vi "Weather Simulator.vi"() -> ()   [LabVIEW 2023]
doc: "The main VI for the Weather Monitor Simulator built application. This VI simulates weather data and puts the simulated data into the Weather Monitor data store, which allows the included web service to access the data."
uses:
  Weather Data.ctl
  Weather Data.lvlib
panel:
  in  "Enable CORS":bool
  in  "Update interval":i32=1000
  out "Wind Direction":dbl
  out "Wind Speed":dbl
  out "Pressure":dbl
  out "Temperature":dbl
  in  "Stop":bool
  # "Overview: Demonstrates the use of Web Services in a built application to provide remote access to an application's data.\nRequirements: LabVIEW Full Development System\nInstructions:\n1. Build and run the Weather Simulator (Server) build specification.\n2. Run the Weather Monitor.vi client or build and run the Weather Monitor (Client) build specification.\n3. See README.htm for more information, including how to run this VI for debugging."
  # "Weather Data Simulator"
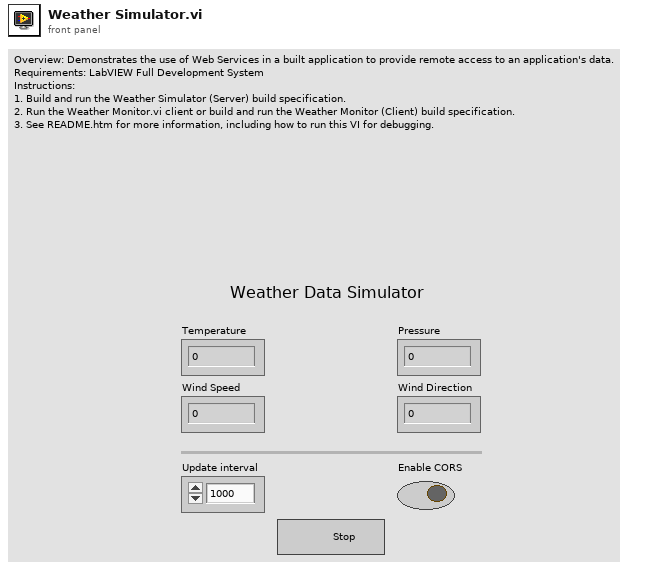
[diagram p1: front panel]
types:
  T1 = typedef "Weather Data.lvlib/Weather Data.ctl" = cluster{"Temperature":dbl, "Pressure":dbl, "Wind Speed":dbl, "Wind Direction":dbl}
  T2 = typedef "Web Service Settings.ctl" = cluster{"Enable CORS":bool}
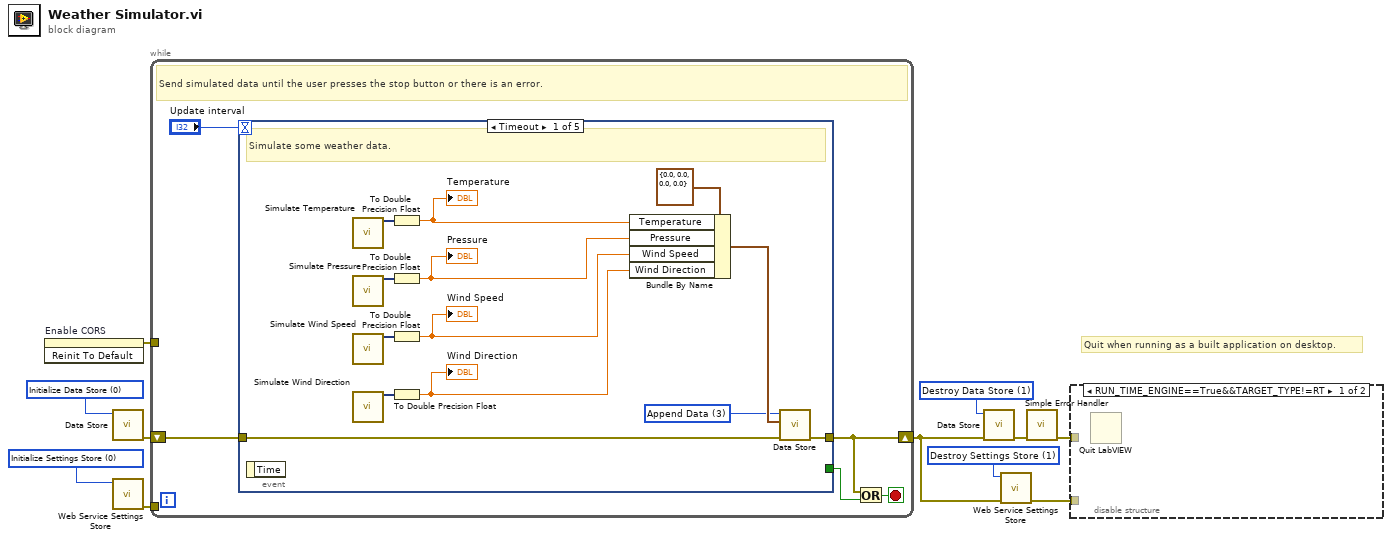
[diagram p0: block diagram]
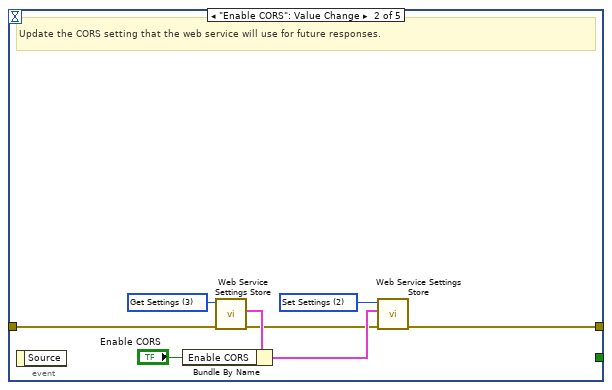
[diagram p3: hidden frame]
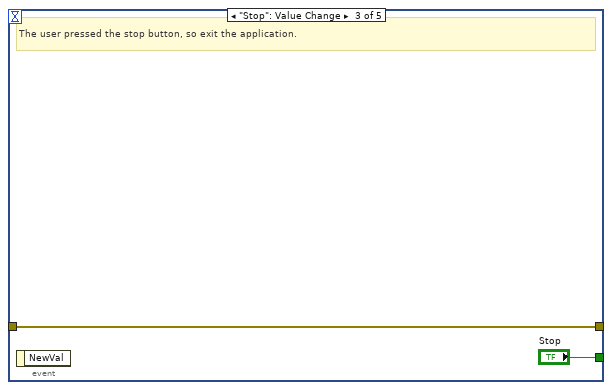
[diagram p4: hidden frame]
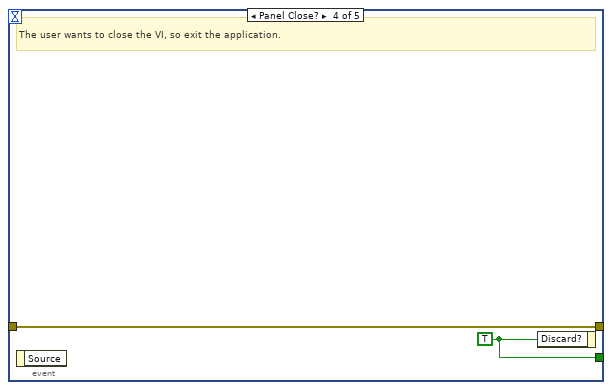
[diagram p5: hidden frame]
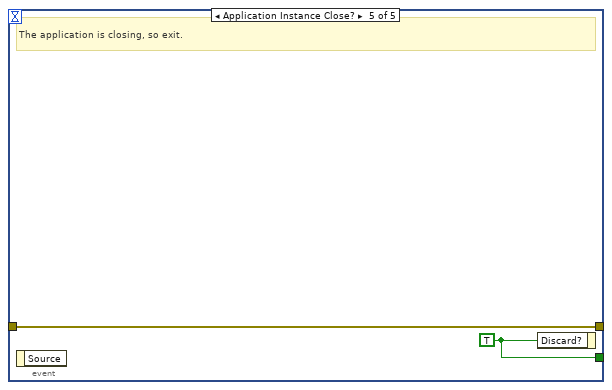
[diagram p6: hidden frame]
diagram:
  w4 = u16 1 items=["Initialize Settings Store", "Destroy Settings Store", "Set Settings", "Get Settings"] ("action")
  w6 = u16 0 items=["Initialize Settings Store", "Destroy Settings Store", "Set Settings", "Get Settings"] ("action")
  w8 = u16 1 items=["Initialize Data Store", "Destroy Data Store", "Clear Data", "Append Data", "Get Last Data", "Get All Data"] ("action")
  w10 = u16 0 items=["Initialize Data Store", "Destroy Data Store", "Clear Data", "Append Data", "Get Last Data", "Get All Data"] ("action")
  # "Quit when running as a built application on desktop."
  n1 = invoke on="Enable CORS" class="Bool (strict)" method="Reinit To Default"() -> (error out=w1:errorcluster)  [unwired: 3 in, 2 out]
  n2 = call "Data Store.vi"("action"=w10) -> ("error out"=w9:errorcluster)  [unwired: 9 in, 1 out]
  n3 = call "Web Service Settings Store.vi"("action"=w6) -> ("error out"=w5:errorcluster)  [unwired: 9 in, 1 out]
  n4 = while {
    shift-right: [w14] -> w3
    shift-left: w9 -> [w16]
    tunnel: w5 -> [_]
    tunnel: w1 -> [_]
    stop <- w15 stop-if-true
    # "Send simulated data until the user presses the stop button or there is an error."
    n5 = event shown="[0] Timeout" {
      selector: _ -> [_ _ _ _ _]
      dyn-events: _ -> [_ _ _ _ _]
      timeout: "Update interval" -> [_ _ _ _ _]
      tunnel: w16 -> [w25 w31 w39 w41 w43]
      tunnel: [w23 w30 w39 w41 w43] -> w14
      tunnel: [_ _ "Stop" w40 w42] -> w12
      event Timeout {
        w17 = u16 3 items=["Initialize Data Store", "Destroy Data Store", "Clear Data", "Append Data", "Get Last Data", "Get All Data"] ("action")
        # "Simulate some weather data."
        n6 = event-data() -> ()  [unwired: 1 in, 1 out]
        n7 = call "Simulate Temperature"() -> ("DC with Uniform Noise"=w22:dynamicdata)  [unwired: 5 in, 10 out]
        n8 = call "Simulate Pressure"() -> ("Sine with Uniform Noise"=w28:dynamicdata)  [unwired: 8 in, 7 out]
        n9 = call "Simulate Wind Speed"() -> ("Sine with Uniform Noise"=w27:dynamicdata)  [unwired: 8 in, 7 out]
        n10 = call "Simulate Wind Direction"() -> ("Sine with Uniform Noise"=w26:dynamicdata)  [unwired: 8 in, 7 out]
        n11 = To Double Precision Float(number=w22) -> (double precision float=w21:dbl)
        "Temperature" <- w21
        n12 = To Double Precision Float(number=w28) -> (double precision float=w20:dbl)
        "Pressure" <- w20
        n13 = To Double Precision Float(number=w27) -> (double precision float=w19:dbl)
        "Wind Speed" <- w19
        n14 = To Double Precision Float(number=w26) -> (double precision float=w18:dbl)
        "Wind Direction" <- w18
        n15 = Bundle By Name(cluster=T1 {"Temperature"=0.0, "Pressure"=0.0, "Wind Speed"=0.0, "Wind Direction"=0.0} ("Weather Data"), "Temperature"=w21, "Pressure"=w20, "Wind Speed"=w19, "Wind Direction"=w18) -> (w24:T1)
        n16 = call "Data Store.vi"("error in (no error)"=w25, "new weather data"=w24, "action"=w17) -> ("error out"=w23:errorcluster)  [unwired: 7 in, 1 out]
      }
      event "Enable CORS": Value Change {
        w34 = u16 2 items=["Initialize Settings Store", "Destroy Settings Store", "Set Settings", "Get Settings"] ("action")
        w37 = u16 3 items=["Initialize Settings Store", "Destroy Settings Store", "Set Settings", "Get Settings"] ("action")
        # "Update the CORS setting that the web service will use for future responses."
        n17 = event-data() -> ()  [unwired: 1 in, 1 out]
        n18 = call "Web Service Settings Store.vi"("error in (no error)"=w31, "action"=w37) -> ("error out"=w32:errorcluster, "settings out"=w36:T2)  [unwired: 8 in]
        n19 = Bundle By Name(cluster=w36, "Enable CORS"="Enable CORS") -> (w33:T2)
        n20 = call "Web Service Settings Store.vi"("error in (no error)"=w32, "new settings"=w33, "action"=w34) -> ("error out"=w30:errorcluster)  [unwired: 7 in, 1 out]
      }
      event "Stop": Value Change {
        # "The user pressed the stop button, so exit the application."
        n21 = event-data() -> ()  [unwired: 1 in, 1 out]
      }
      event Panel Close? {
        w40 = TRUE ("Discard?")
        # "The user wants to close the VI, so exit the application."
        n22 = event-data() -> ()  [unwired: 1 in, 1 out]
        n23 = event-data("Discard?"=w40) -> ()  [unwired: 1 in, 1 out]
      }
      event Application Instance Close? {
        w42 = TRUE ("Discard?")
        # "The application is closing, so exit."
        n24 = event-data() -> ()  [unwired: 1 in, 1 out]
        n25 = event-data("Discard?"=w42) -> ()  [unwired: 1 in, 1 out]
      }
    }
    n26 = Or(x=w14, y=w12) -> (x .or. y?=w15:bool)
  }
  n27 = call "Data Store.vi"("error in (no error)"=w3, "action"=w8) -> ("error out"=w11:errorcluster)  [unwired: 8 in, 1 out]
  n28 = call "Web Service Settings Store.vi"("error in (no error)"=w3, "action"=w4) -> ("error out"=w2:errorcluster)  [unwired: 8 in, 1 out]
  n29 = call <vilib>:"Simple Error Handler.vi"("error in (no error)"=w11) -> ("error out"=w7:errorcluster)  [unwired: 4 in, 4 out]
  n30 = disable-structure shown="RUN_TIME_ENGINE==True&&TARGET_TYPE!=RT" {
    disable-tunnel: w7 -> [_ _]
    disable-tunnel: w2 -> [_ _]
    frame condition #0 {
      n31 = Quit LabVIEW() -> ()  [unwired: 1 in]
    }
    frame condition #1 (active) {
    }
  }
